vi "Int32Array Create (Dimensions).vi"(8 "error in (no error)":errorcluster, 10 "Array dimensions":i32[](array[numeric]), 11 "I32 array in":i32[](array[numeric])) -> (0 "error out":errorcluster, 3 "Int32Array DVR out":refnum<data-value>)   [LabVIEW 2010, in "MDSplus.lvlib"]
uses:
  <vilib>/MDSplus/Library/MDSplus.lvlib
  <vilib>/MDSplus/Classes/Data_Class/Array_Class/Int32Array_Class/Int32Array.lvclass
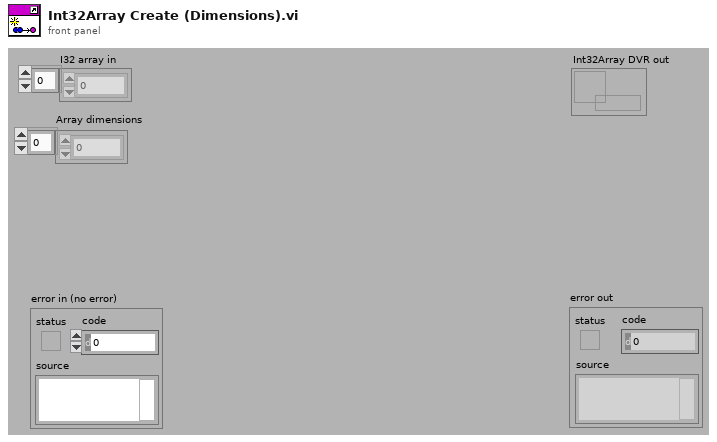
[diagram p1: front panel]
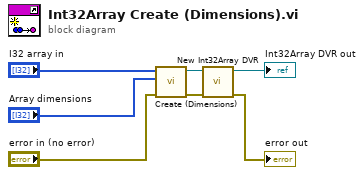
[diagram p0: block diagram]
diagram:
  n1 = call <vilib>:"Create (Dimensions).vi"("error in (no error)"="error in (no error)", "Dimensions"="Array dimensions", "I32 array in"="I32 array in") -> ("error out"=w4:errorcluster, "Int32Array out"=w5:refnum<class "Int32Array.lvclass">)  [unwired: 7 in]
  n2 = call <vilib>:"New Int32Array DVR.vi"("error in (no error)"=w4, "Int32Array in"=w5) -> ("error out"=→"error out":errorcluster, "Int32Array DVR out"=→"Int32Array DVR out":refnum<data-value>)  [unwired: 8 in]
